vi "Get XNET Signal Names.vi"(6 "Add Info?":bool, 7 "Parent Ref in":T1 format="%.0x", 8 "error in":errorcluster, 9 "Tree In":refnum<vi>, 10 "Parent":string, 11 "Frms":refnum<k21>[](array[refnum])) -> (0 "error out":errorcluster, 1 "Tree Out":refnum<vi>, 3 "XNET Signal Names":refnum<k21>[](array[refnum]))   [LabVIEW 2015, in "J1939 Addon System Explorer.lvlib"]
uses:
  J1939 Addon System Explorer.lvlib
  <vilib>/NI Veristand/Custom Device API/Custom Device Item Ref.ctl
  <vilib>/NI Veristand/Custom Device API/Custom Device Channel.ctl
  <vilib>/NI Veristand/Custom Device API/Custom Device Channel Type.ctl
  Shared/Types/SPN Properties.ctl
  Shared/SubVIs/Constants.vi
  <vilib>/NI Veristand/Custom Device API/Set Item Property (U32).vi
  <resource>/objmgr/xnet.rc
  <vilib>/NI VeriStand/Custom Device API/Custom Device API.lvlib
  Shared/J1939 Addon Shared.lvlib
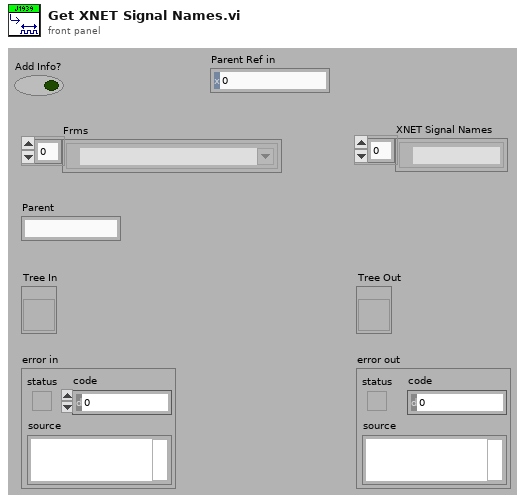
[diagram p1: front panel]
types:
  T1 = typedef "Custom Device API.lvlib/Custom Device Item Ref.ctl" = u64
  T2 = typedef "Custom Device API.lvlib/Custom Device Channel.ctl" = cluster{"Type":T3, "Units":string, "Default Value":dbl, "Faultable":bool, "Scalable":bool}
  T3 = typedef "Custom Device API.lvlib/Custom Device Channel Type.ctl" = enum16{"Input", "Output"}
  T4 = typedef "J1939 Addon Shared.lvlib/SPN Properties.ctl" = cluster{"Bytes":u32, "ScaleFac":dbl, "ScaleOff":dbl}
  T5 = typedef "Custom Device API.lvlib/Custom Device Item Info.ctl" = cluster{"Name":string, "Is Channel":bool, "GUID":string, "Is Waveform":bool}
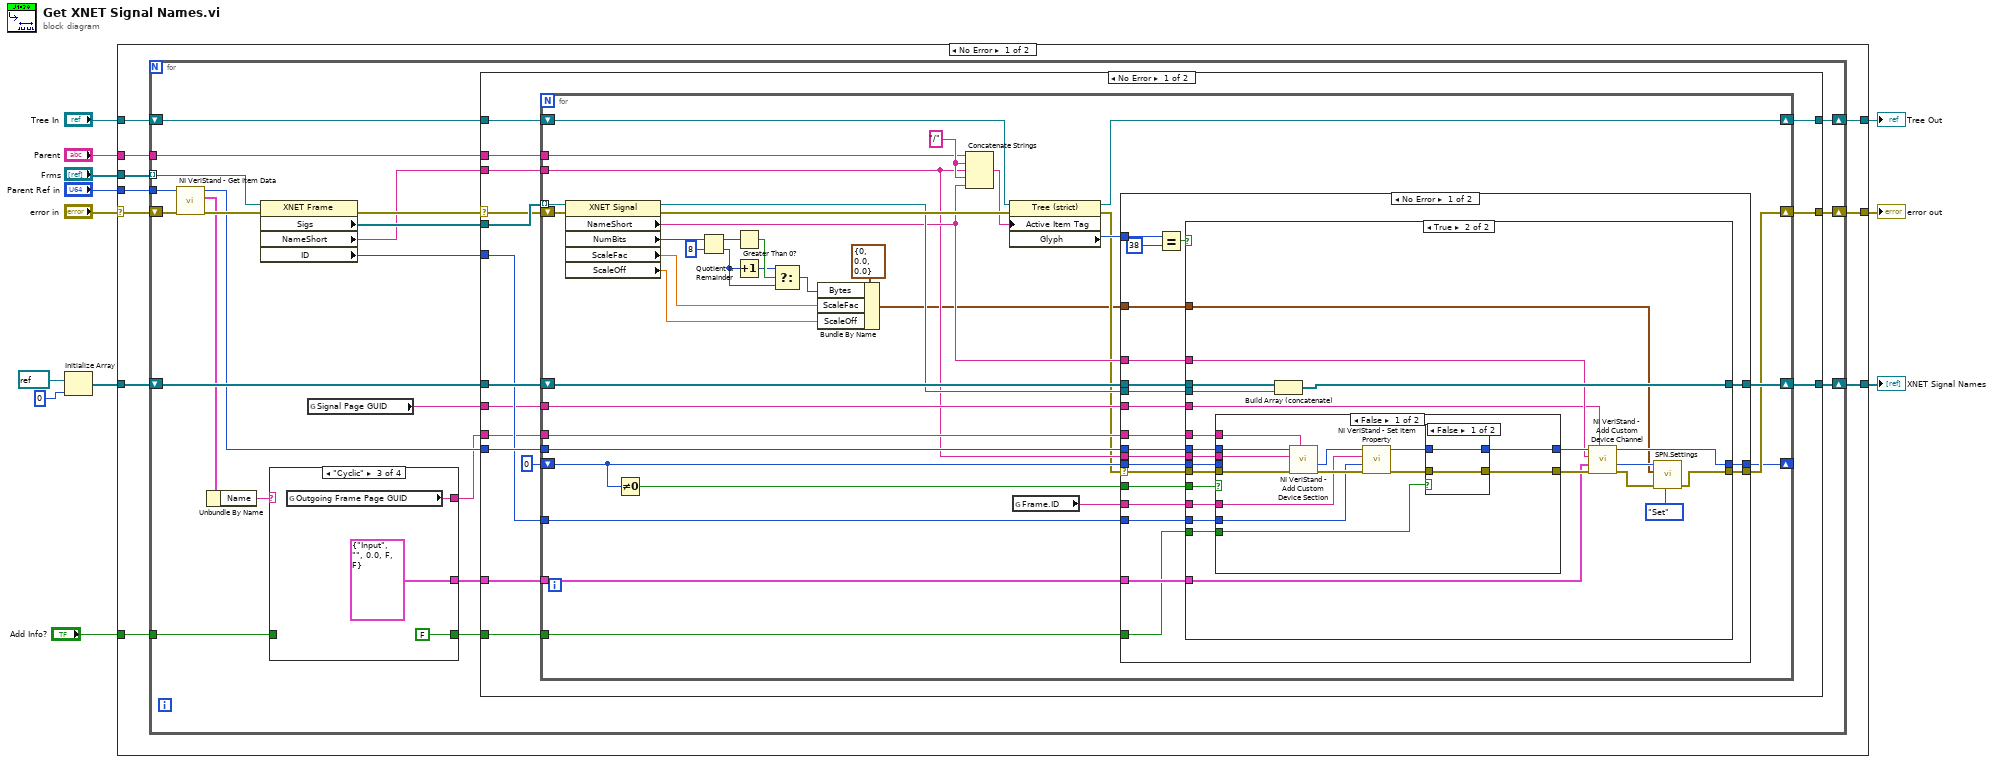
[diagram p0: block diagram]
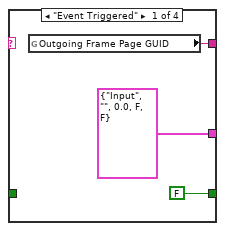
[diagram p2: hidden frame]
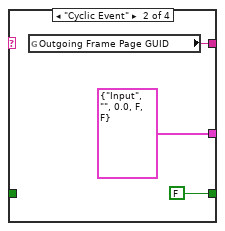
[diagram p3: hidden frame]
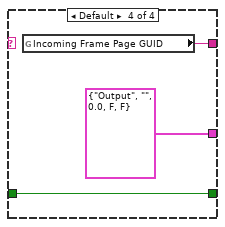
[diagram p4: hidden frame]
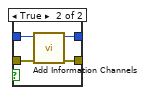
[diagram p6: hidden frame]
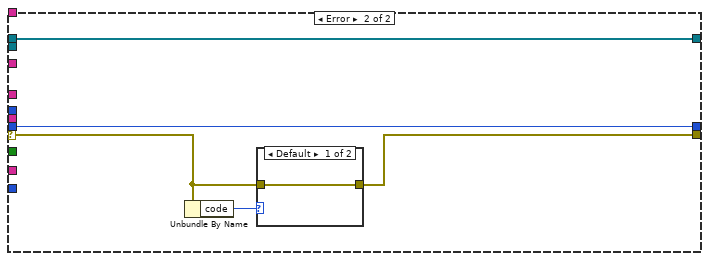
[diagram p8: hidden frame]
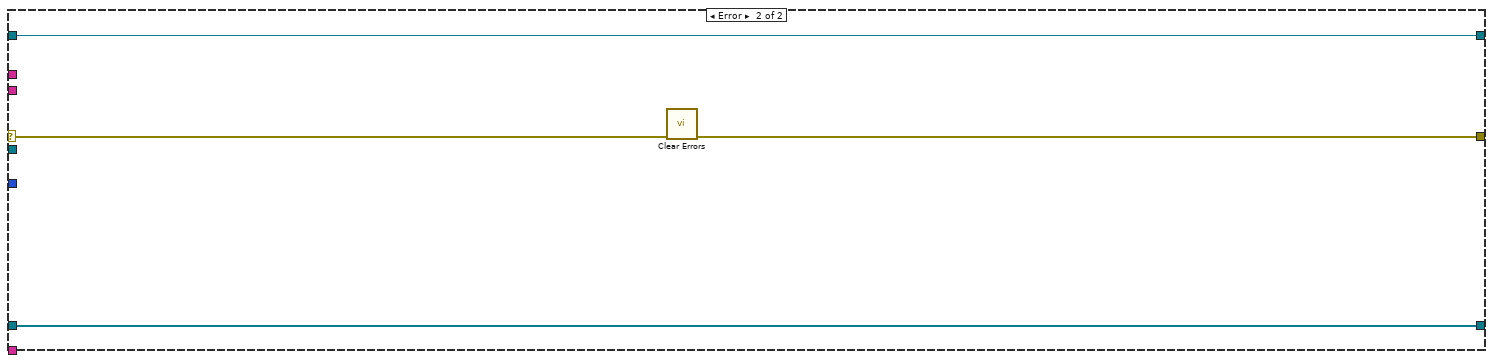
[diagram p10: hidden frame]
diagram:
  n1 = Initialize Array(refnum<k21> refnum ("XNET Signal"), 0 ("dimension size")) -> (w6:refnum<k21>[])
  n2 = case shown="No Error" "error in" {
    selector: "error in" -> [w19 w189]
    tunnel: "Parent" -> [w22 _]
    tunnel: [w21 w189] -> w11
    tunnel: "Frms" -> [w20 _]
    tunnel: [w18 _] -> w8
    tunnel: w6 -> [w17 _]
    tunnel: "Tree In" -> [w16 w188]
    tunnel: [w15 w188] -> w3
    tunnel: "Parent Ref in" -> [w14 _]
    tunnel: "Add Info?" -> [w13 _]
    frame No Error {
      n3 = for {
        shift-right: [w41] -> w21
        shift-left: w19 -> [w35]
        tunnel: w20 -> [w44] mode=indexing
        tunnel: w22 -> [w42]
        shift-right: [w38] -> w18
        shift-left: w17 -> [w39]
        shift-right: [w37] -> w15
        shift-left: w16 -> [w40]
        tunnel: w14 -> [w33]
        tunnel: w13 -> [w26]
        n4 = call <vilib>:"NI VeriStand - Get Item Data.vi"("error in (no error)"=w35, "Item Ref in"=w33) -> ("error out"=w34:errorcluster, "Item Info"=w31:T5, "Item Ref out"=w32:T1)  [unwired: 7 out]
        n5 = Unbundle By Name(w31) -> ("Name"=w30:string)
        n6 = property class="XNET Frame"(reference=w44, error in=w34) -> (error out=w36:errorcluster, "Sigs"=w43:refnum<k21>[], "NameShort"=w28:string, "ID"=w27:u32)  [unwired: 1 out]
        n7 = case shown="\"Cyclic\"" w30 {
          tunnel: [T2 {"Type"=enum."Input", "Units"="", "Default Value"=0.0, "Faultable"=FALSE, "Scalable"=FALSE} ("Channel") T2 {"Type"=enum."Input", "Units"="", "Default Value"=0.0, "Faultable"=FALSE, "Scalable"=FALSE} ("Channel") T2 {"Type"=enum."Input", "Units"="", "Default Value"=0.0, "Faultable"=FALSE, "Scalable"=FALSE} ("Channel") T2 {"Type"=enum."Output", "Units"="", "Default Value"=0.0, "Faultable"=FALSE, "Scalable"=FALSE} ("Channel")] -> w29
          tunnel: [FALSE ("Add Info?") FALSE ("Add Info?") FALSE ("Add Info?") w55] -> w25
          tunnel: w26 -> [_ _ _ w55]
          tunnel: [w45 w48 w51 w54] -> w23
          frame "Event Triggered" {
            n8 = global read "Constants.vi" "Outgoing Frame Page GUID"() -> (w45:string)
          }
          frame "Cyclic Event" {
            n9 = global read "Constants.vi" "Outgoing Frame Page GUID"() -> (w48:string)
          }
          frame "Cyclic" {
            n10 = global read "Constants.vi" "Outgoing Frame Page GUID"() -> (w51:string)
          }
          frame Default {
            n11 = global read "Constants.vi" "Incoming Frame Page GUID"() -> (w54:string)
          }
        }
        n12 = global read "Constants.vi" "Signal Page GUID"() -> (w24:string)
        n13 = case shown="No Error" w36 {
          selector: w36 -> [w62 w184]
          tunnel: w43 -> [w72 _]
          tunnel: w28 -> [w71 _]
          tunnel: w42 -> [w70 _]
          tunnel: [w69 w185] -> w41
          tunnel: w40 -> [w68 w186]
          tunnel: w39 -> [w67 w187]
          tunnel: [w66 w187] -> w38
          tunnel: [w65 w186] -> w37
          tunnel: w32 -> [w64 _]
          tunnel: w27 -> [w61 _]
          tunnel: w24 -> [w60 _]
          tunnel: w23 -> [w59 _]
          tunnel: w29 -> [w58 _]
          tunnel: w25 -> [w57 _]
          frame No Error {
            n14 = for {
              tunnel: w72 -> [w109] mode=indexing
              tunnel: w71 -> [w86]
              tunnel: w70 -> [w106]
              shift-right: [w97] -> w69
              shift-left: w62 -> [w108]
              shift-right: [w101] -> w66
              shift-left: w67 -> [w100]
              shift-right: [w98] -> w65
              shift-left: w68 -> [w104]
              tunnel: w64 -> [w96]
              shift-right: [w95] -> _
              shift-left: T1 0 ("Parent Ref out") -> [w94]
              tunnel: w61 -> [w91]
              tunnel: w60 -> [w89]
              tunnel: w59 -> [w88]
              tunnel: w58 -> [w87]
              tunnel: w57 -> [w74]
              w107 = "/" ("string")
              n15 = property class="XNET Signal"(reference=w109, error in=w108) -> (reference out=w99:refnum<k21>, error out=w105:errorcluster, "NameShort"=w92:string, "NumBits"=w85:u32, "ScaleFac"=w78:dbl, "ScaleOff"=w77:dbl)
              n16 = Not Equal To 0?(x=w94) -> (x != 0?=w93:bool)
              n17 = Quotient & Remainder(x=w85, y=u32 8) -> (x-y*floor(x/y)=w83:u32, floor(x/y)=w81:u32)
              n18 = Greater Than 0?(x=w83) -> (x > 0?=w82:bool)
              n19 = Increment(x=w81) -> (x+1=w80:u32)
              n20 = Select(t=w80, s=w82, f=w81) -> (s? t:f=w79:u32)
              n21 = Bundle By Name(cluster=T4 {"Bytes"=0, "ScaleFac"=0.0, "ScaleOff"=0.0}, "Bytes"=w79, "ScaleFac"=w78, "ScaleOff"=w77) -> (w73:T4)
              n22 = Concatenate Strings(w106, w107, w86, w107, w92) -> (w103:string)
              n23 = property class="Tree (strict)"(reference=w104, error in=w105, "Active Item Tag"=w103) -> (reference out=w98:refnum<vi>, error out=w75:errorcluster, "Glyph"=w102:i32)
              n24 = global read "Constants.vi" "Frame.ID"() -> (w90:string)
              n25 = case shown="No Error" w75 {
                selector: w75 -> [w111 w179]
                tunnel: w102 -> [w130 _]
                tunnel: [w127 w181] -> w101
                tunnel: w100 -> [w126 w181]
                tunnel: w99 -> [w125 _]
                tunnel: [w124 w178] -> w97
                tunnel: w96 -> [w123 _]
                tunnel: [w122 w182] -> w95
                tunnel: w94 -> [w121 w182]
                tunnel: w93 -> [w120 _]
                tunnel: w92 -> [w119 _]
                tunnel: w91 -> [w118 _]
                tunnel: w90 -> [w117 _]
                tunnel: w89 -> [w116 _]
                tunnel: w88 -> [w115 _]
                tunnel: w87 -> [w114 _]
                tunnel: w86 -> [w113 _]
                tunnel: w73 -> [w112 _]
                tunnel: w74 -> [w110 _]
                frame No Error {
                  n26 = Equal?(x=w130, y=38) -> (x = y?=w128:bool)
                  n27 = case shown="True" w128 {
                    tunnel: [w133 w154] -> w127
                    tunnel: w126 -> [w133 w156]
                    tunnel: w125 -> [_ w155]
                    tunnel: w120 -> [_ w153]
                    tunnel: w113 -> [_ w152]
                    tunnel: w111 -> [w132 w151]
                    tunnel: [w132 w136] -> w124
                    tunnel: w123 -> [_ w150]
                    tunnel: [w131 w147] -> w122
                    tunnel: w121 -> [w131 w149]
                    tunnel: w119 -> [_ w145]
                    tunnel: w115 -> [_ w144]
                    tunnel: w116 -> [_ w143]
                    tunnel: w118 -> [_ w142]
                    tunnel: w117 -> [_ w141]
                    tunnel: w114 -> [_ w140]
                    tunnel: w112 -> [_ w134]
                    tunnel: w110 -> [_ w139]
                    frame False {
                    }
                    frame True {
                      n28 = case shown="False" w153 {
                        tunnel: w152 -> [w169 _]
                        tunnel: w151 -> [w168 w177]
                        tunnel: [w163 w177] -> w148
                        tunnel: w150 -> [w167 _]
                        tunnel: [w162 w176] -> w146
                        tunnel: w149 -> [_ w176]
                        tunnel: w144 -> [w166 _]
                        tunnel: w142 -> [w157 _]
                        tunnel: w141 -> [w158 _]
                        tunnel: w139 -> [w164 _]
                        frame False {
                          n29 = call <vilib>:"NI VeriStand - Add Custom Device Section.vi"("GUID (Default Section)"=w166, "error in (no error)"=w168, "Section Name"=w169, "Parent Ref in"=w167) -> ("error out"=w160:errorcluster, "Section Ptr"=w165:T1)  [unwired: 4 in, 2 out]
                          n30 = call-poly <vilib>:"NI VeriStand - Set Item Property.vi"("error in (no error)"=w160, "Value"=w157, "Property Name"=w158, "Item Ref in"=w165) -> ("error out"=w159:errorcluster, "Item Ref out"=w161:T1)  [unwired: 5 in, 1 out]
                          n31 = case shown="False" w164 {
                            tunnel: w161 -> [w170 w175]
                            tunnel: [w170 w174] -> w162
                            tunnel: w159 -> [w171 w173]
                            tunnel: [w171 w172] -> w163
                            frame False {
                            }
                            frame True {
                              n32 = call "Add Information Channels.vi"("error in (no error)"=w173, "Node Ptr"=w175) -> ("error out"=w172:errorcluster, "Parent Ref out"=w174:T1)  [unwired: 8 in]
                            }
                          }
                        }
                        frame True {
                        }
                      }
                      n33 = Build Array (concatenate)(w156, w155) -> (w154:refnum<k21>[])
                      n34 = call <vilib>:"NI VeriStand - Add Custom Device Channel.vi"("GUID (Default Channel)"=w143, "error in (no error)"=w148, "Channel"=w140, "Channel Name"=w145, "Parent Ref in"=w146) -> ("error out"=w137:errorcluster, "Channel Ref"=w138:T1, "Parent Ref out"=w147:T1)  [unwired: 3 in, 1 out]
                      n35 = call "SPN.Settings.vi"("Action"=enum8{"Get", "Set"}."Set", "error in (no error)"=w137, "SPN.Settings"=w134, "Item Ref in"=w138) -> ("error out"=w136:errorcluster)  [unwired: 5 in, 2 out]
                    }
                  }
                }
                frame Error {
                  n36 = Unbundle By Name(w179) -> ("code"=w180:i32)
                  n37 = case shown="Default" w180 {
                    tunnel: [w183 _] -> w178
                    tunnel: w179 -> [w183 _]
                    frame Default {
                    }
                    frame 1136 {
                    }
                  }
                }
              }
            }
          }
          frame Error {
            n38 = call <vilib>:"Clear Errors.vi"("error in (no error)"=w184) -> ("error out"=w185:errorcluster)  [unwired: 5 in, 1 out]
          }
        }
      }
    }
    frame Error {
    }
  }
  "error out" <- w11
  "XNET Signal Names" <- w8
  "Tree Out" <- w3
